vi "Omni-Driver-Fast-Acquire.vi"(4 "Correct Electrical Dark":bool=TRUE, 5 "Spectrometer number":i32, 6 "Integration Time (ms)":i32=100, 7 "Wrapper":u32) -> (0 "Length":i32, 1 "Spectrum Values":dbl[](array[numeric]), 2 "WL Values":dbl[](array[numeric]), 3 "Wrapper Out":u32)   [LabVIEW 2014]
doc: "André Romero - 2016\nandretec@ifsc.usp.br"
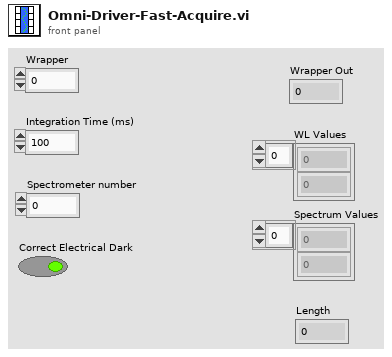
[diagram p1: front panel]
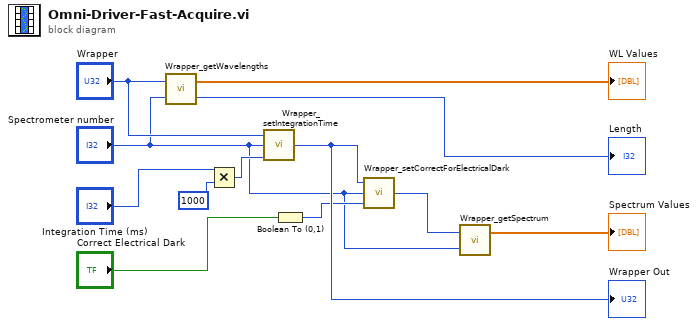
[diagram p0: block diagram]
diagram:
  n1 = call "Wrapper_getWavelengths.vi"("Index"="Spectrometer number", "Wrapper"="Wrapper") -> ("Length"=→"Length":i32, "WL Values"=→"WL Values":dbl[])
  n2 = Multiply(x="Integration Time (ms)", y=1000) -> (x*y=w12:i32)
  n3 = call "Wrapper_setIntegrationTime.vi"("Integration Time"=w12, "Index"="Spectrometer number", "Wrapper In"="Wrapper") -> ("Wrapper Out"=w6:u32)
  "Wrapper Out" <- w6
  n4 = Boolean To (0,1)(Boolean="Correct Electrical Dark") -> (0, 1=w5:i16)
  n5 = call "Wrapper_setCorrectForElectricalDark.vi"("On/Off"=w5, "Index"="Spectrometer number", "Wrapper In"=w6) -> ("Wrapper Out"=w2:u32)
  n6 = call "Wrapper_getSpectrum.vi"("Index"="Spectrometer number", "Wrapper"=w2) -> ("Spectrum Values"=→"Spectrum Values":dbl[])  [unwired: 1 out]
